vi "Timer FGV.vi"(7 "Action":T1, 8 "error in (no error)":errorcluster) -> (0 "error out":errorcluster, 3 "Elapsed Time":dbl)   [LabVIEW 2015]
uses:
  Timer Actions.ctl
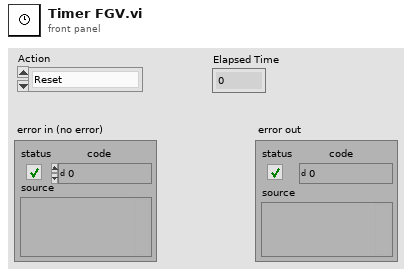
[diagram p1: front panel]
types:
  T1 = typedef "Timer Actions.ctl" = enum16{"Reset", "Get"}
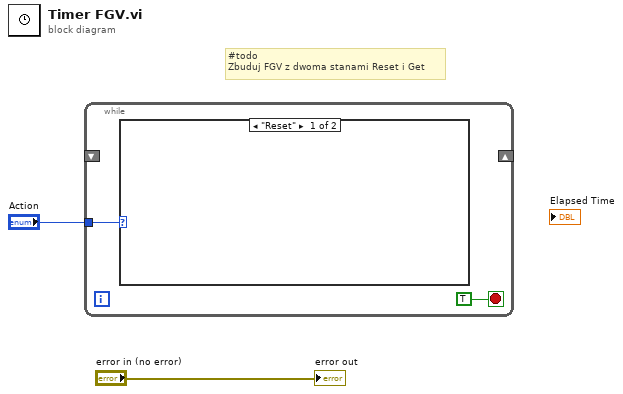
[diagram p0: block diagram]
diagram:
  # "#todo \nZbuduj FGV z dwoma stanami Reset i Get"
  n1 = while {
    shift-right: _ -> [_]
    shift-left: _ -> [_]
    tunnel: "Action" -> [w3]
    stop <- TRUE stop-if-true
    n2 = case shown="\"Reset\"" w3 {
      frame "Reset" {
      }
      frame "Get" {
      }
    }
  }
  "error out" <- "error in (no error)"
